vi "ConfigureDifferentialMP.vi"(10 "Right Side":T1, 11 "Left Side":T1) -> (2 "Right Side":T1, 3 "Left Side":T1)   [LabVIEW 2017]
uses:
  <vilib>/Rock Robotics/WPI/MotorControl/WPI_MotorControlDeviceRef.ctl
  <vilib>/Rock Robotics/WPI/MotorControl/WPI_MotorControlType.ctl
  <vilib>/Rock Robotics/SystemInterfaces/DIO/FPGA_DIOPWMChannel.ctl
  <vilib>/Rock Robotics/WPI/PWM/WPI_PWMDeadband.ctl
  <vilib>/Rock Robotics/SystemInterfaces/DIO/FPGA_DIOChannel.ctl
  <vilib>/Rock Robotics/WPI/ThirdParty/Phoenix-LabVIEW/Motor Controller/Controls/CTRE_Phoenix_MotorControl_FeedbackDevice.ctl
  <vilib>/Rock Robotics/WPI/ThirdParty/Phoenix-LabVIEW/Motor Controller/Controls/CTRE_Phoenix_MotorControl_RemoteSourceType.ctl
  <vilib>/Rock Robotics/WPI/ThirdParty/Phoenix-LabVIEW/Motor Controller/Controls/CTRE_Phoenix_MotorControl_SensorTermFeedbackDevice_Enhanced.ctl
  <vilib>/Rock Robotics/WPI/ThirdParty/Phoenix-LabVIEW/Motor Controller/Controls/CTRE_Phoenix_MotorControl_StatusFrameEnhanced.ctl
  <vilib>/Rock Robotics/WPI/ThirdParty/Phoenix-LabVIEW/Motor Controller/Controls/CTRE_Phoenix_MotorControl_NeutralMode.ctl
  <vilib>/Rock Robotics/WPI/ThirdParty/Phoenix-LabVIEW/Motor Controller/Controls/CTRE_Phoenix_MotorControl_ControlMode.ctl
  <vilib>/Rock Robotics/WPI/ThirdParty/Phoenix-LabVIEW/Controls/CTRE_Phoenix_Params.ctl
  Constants.vi
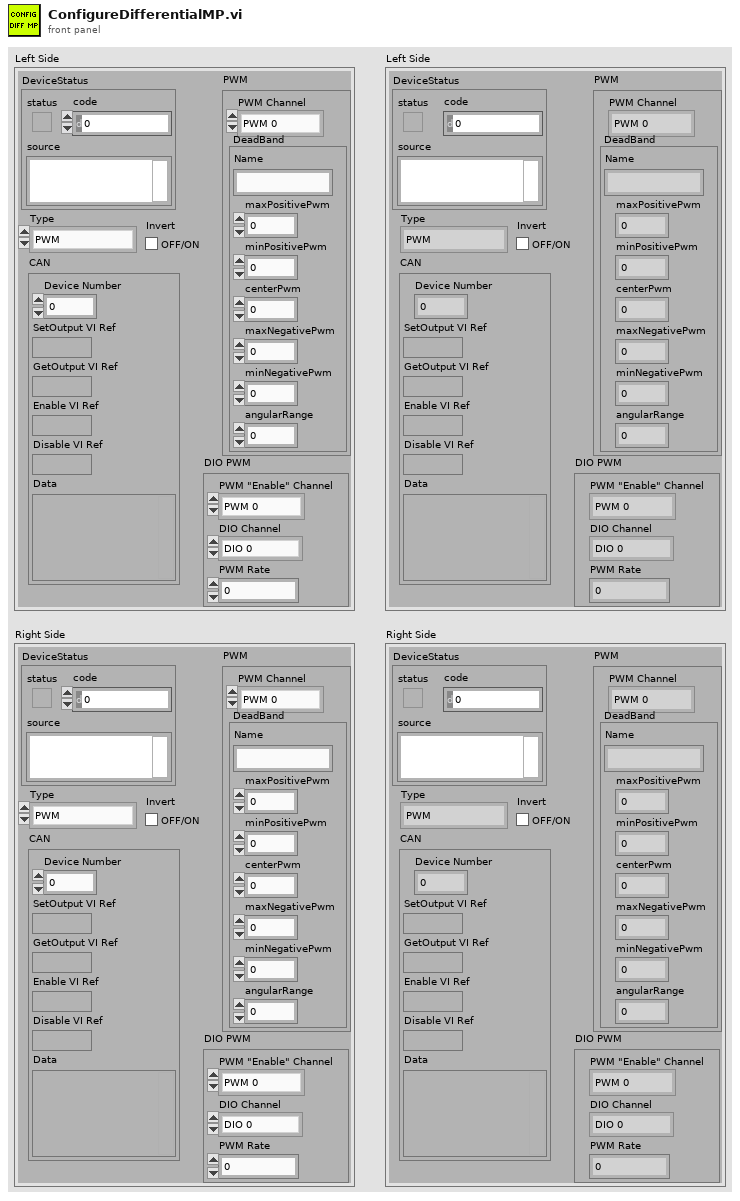
[diagram p1: front panel]
types:
  T1 = typedef "WPI_MotorControlDeviceRef.ctl" = cluster{"DeviceStatus":errorcluster, "Type":T2, "PWM":cluster{"PWM Channel":T3, "DeadBand":T4}, "CAN":cluster{"Device Number":u8, "SetOutput VI Ref":variant, "GetOutput VI Ref":variant, "Enable VI Ref":variant, "Disable VI Ref":variant, "Data":variant}, "Invert":bool, "DIO PWM":cluster{"PWM \"Enable\" Channel":T3, "DIOChannel":T5, "PWM Rate":dbl}}
  T2 = typedef "WPI_MotorControlType.ctl" = enum16{"PWM", "CAN", "DIO PWM"}
  T3 = typedef "FPGA_DIOPWMChannel.ctl" = enum8{"PWM 0", "PWM 1", "PWM 2", "PWM 3", "PWM 4", "PWM 5", "PWM 6", "PWM 7", "PWM 8", "PWM 9", "PWM MXP 0", "PWM MXP 1", "PWM MXP 2", "PWM MXP 3", "PWM MXP 4", "PWM MXP 5", "PWM MXP 6", "PWM MXP 7", "PWM MXP 8", "PWM MXP 9", "Invalid"}
  T4 = typedef "WPI_PWMDeadband.ctl" = cluster{"Name":string, "maxPositivePwm":i32, "minPositivePwm":i32, "centerPwm":i32, "maxNegativePwm":i32, "minNegativePwm":i32, "angularRange":u16}
  T5 = typedef "FPGA_DIOChannel.ctl" = enum8{"DIO 0", "DIO 1", "DIO 2", "DIO 3", "DIO 4", "DIO 5", "DIO 6", "DIO 7", "DIO 8", "DIO 9", "DIO MXP 0", "DIO MXP 1", "DIO MXP 2", "DIO MXP 3", "DIO MXP 4", "DIO MXP 5", "DIO MXP 6", "DIO MXP 7", "DIO MXP 8", "DIO MXP 9", "DIO MXP 10", "DIO MXP 11", "DIO MXP 12", "DIO MXP 13", "DIO MXP 14", "DIO MXP 15", "SPI Port CS1", "SPI Port CS2", "SPI Port CS3", "SPI Port MISO", "SPI Port MOSI", "Invalid"}
  T6 = typedef "CTRE_Phoenix_Params.ctl" = u16
  T7 = typedef "CTRE_Phoenix_MotorControl_ControlMode.ctl" = u16
  T8 = typedef "CTRE_Phoenix_MotorControl_NeutralMode.ctl" = enum8{"EEPROMSetting", "Override to Coast", "Override to Brake"}
  T9 = typedef "CTRE_Phoenix_MotorControl_StatusFrameEnhanced.ctl" = u16
  T10 = typedef "CTRE_Phoenix_MotorControl_FeedbackDevice.ctl" = i8
  T11 = typedef "CTRE_Phoenix_MotorControl_SensorTermFeedbackDevice_Enhanced.ctl" = i8
  T12 = typedef "CTRE_Phoenix_MotorControl_RemoteSourceType.ctl" = enum16{"Off", "Talon SRX Selected Sensor", "Pigeon IMU Yaw", "Pigeon IMU Pitch", "Pigeon IMU Roll", "CANifier Quadrature", "CANifier PWM Input 0", "CANifier PWM Input 1", "CANifier PWM Input 2", "CANifier PWM Input 3", "Gadgeteer Pigeon Yaw", "Gadgeteer Pigeon Pitch", "Gadgeteer Pigeon Roll"}
  T13 = cluster{"kP":dbl, "kI ":dbl, "kD":dbl, "kF":dbl, "I Zone":dbl, "Peak Out":dbl}
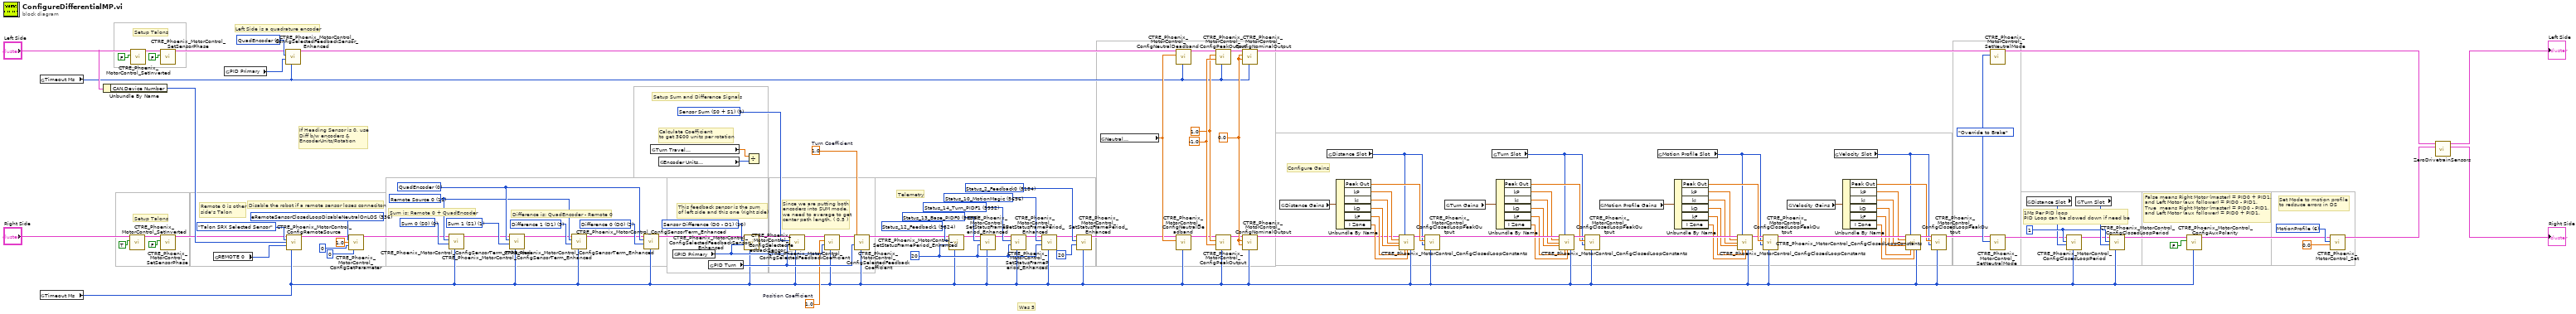
[diagram p0: block diagram]
diagram:
  w1 = 1.0  # Turn Coefficient
  w7 = T6 336 items=["eOnBoot_BrakeMode"=31, "eQuadFilterEn"=91, "eQuadIdxPolarity"=108, "eClearPositionOnIdx"=100, "eMotionProfileHasUnderrunErr"=119, "eMotionProfileTrajectoryPointDurationMs"=120, "eClearPosOnLimitF"=144, "eClearPosOnLimitR"=145, "eStatusFramePeriod"=300, "eOpenLoopRamp"=301, "eClosedLoopRamp"=302, "eNeutralDeadband"=303, "ePeakPosOutput"=305, "eNominalPosOutput"=306, "ePeakNegOutput"=307, "eNominalNegOutput"=308, "eProfileParamSlot_P"=310, "eProfileParamSlot_I"=311, "eProfileParamSlot_D"=312, "eProfileParamSlot_F"=313, "eProfileParamSlot_IZone"=314, "eProfileParamSlot_AllowableErr"=315, "eProfileParamSlot_MaxIAccum"=316, "eClearPositionOnLimitF"=320, "eClearPositionOnLimitR"=321, "eClearPositionOnQuadIdx"=322, "eSampleVelocityPeriod"=325, "eSampleVelocityWindow"=326, "eFeedbackSensorType"=330, "eSelectedSensorPosition"=331, "eFeedbackNotContinuous"=332, "eRemoteSensorSource"=333, "eRemoteSensorDeviceID"=334, "eSensorTerm"=335, "eRemoteSensorClosedLoopDisableNeutralOnLOS"=336, "eForwardSoftLimitThreshold"=340, "eReverseSoftLimitThreshold"=341, "eForwardSoftLimitEnable"=342, "eReverseSoftLimitEnable"=343, "eNominalBatteryVoltage"=350, "eBatterVoltageFilterSize"=351, "eContinuousCurrentLimitAmps"=360, "eContinuousCurrentLimitMs"=361, "ePeakCurrentLimitAmps"=362, "eClosedLoopIAccum"=370, "eCustomParam"=380, "eStickyFaults"=390, "eAnalogPosition"=400, "eQuadraturePosition"=401, "ePulseWidthPosition"=402, "eMotMag_Accel"=410, "eMotMag_VelCruise"=411, "eLimitSwitchSource"=421, "eLimitSwitchNormClosedAndDis"=422, "eLimitSwitchDisabledNeutralOnLOS"=423, "eLimitSwitchRemoteDevID"=424] ("Parameter")
  w20 = T7 6 items=["PercentOutput"=0, "Position"=1, "Velocity"=2, "Current"=3, "Follower"=5, "MotionProfile"=6, "MotionMagic"=7, "MotionProfileArc"=10, "Disabled"=15] ("Control Mode")
  w120 = 1 ("loopTimeMs")
  w116 = CTRE_Phoenix_MotorControl_NeutralMode."Override to Brake" ("Motor Control Neutral Mode")
  w77 = 0.0 ("Forward Nominal Percent Output")
  w74 = -1.0 ("Reverse Peak Percent Output")
  w73 = 1.0 ("Forward Peak Percent Output")
  w16 = 20 ("periodMs")
  w66 = T9 5184 items=["Status_1_General"=5120, "Status_2_Feedback0"=5184, "Status_3_Quadrature"=5248, "Status_4_AinTempVbat"=5312, "Status_6_Misc"=5440, "Status_7_CommStatus"=5504, "Status_8_PulseWidth"=5568, "Status_9_MotProfBuffer"=5632, "Status_10_MotionMagic"=5696, "Status_11_UartGadgeteer"=5760, "Status_12_Feedback1"=5824, "Status_13_Base_PIDF0"=5888, "Status_14_Turn_PIDF1"=5952, "Status_15_FirmwareApiStatus"=6016] ("Status Frame")
  w65 = T9 5696 items=["Status_1_General"=5120, "Status_2_Feedback0"=5184, "Status_3_Quadrature"=5248, "Status_4_AinTempVbat"=5312, "Status_6_Misc"=5440, "Status_7_CommStatus"=5504, "Status_8_PulseWidth"=5568, "Status_9_MotProfBuffer"=5632, "Status_10_MotionMagic"=5696, "Status_11_UartGadgeteer"=5760, "Status_12_Feedback1"=5824, "Status_13_Base_PIDF0"=5888, "Status_14_Turn_PIDF1"=5952, "Status_15_FirmwareApiStatus"=6016] ("Status Frame")
  w64 = T9 5952 items=["Status_1_General"=5120, "Status_2_Feedback0"=5184, "Status_3_Quadrature"=5248, "Status_4_AinTempVbat"=5312, "Status_6_Misc"=5440, "Status_7_CommStatus"=5504, "Status_8_PulseWidth"=5568, "Status_9_MotProfBuffer"=5632, "Status_10_MotionMagic"=5696, "Status_11_UartGadgeteer"=5760, "Status_12_Feedback1"=5824, "Status_13_Base_PIDF0"=5888, "Status_14_Turn_PIDF1"=5952, "Status_15_FirmwareApiStatus"=6016] ("Status Frame")
  w63 = T9 5888 items=["Status_1_General"=5120, "Status_2_Feedback0"=5184, "Status_3_Quadrature"=5248, "Status_4_AinTempVbat"=5312, "Status_6_Misc"=5440, "Status_7_CommStatus"=5504, "Status_8_PulseWidth"=5568, "Status_9_MotProfBuffer"=5632, "Status_10_MotionMagic"=5696, "Status_11_UartGadgeteer"=5760, "Status_12_Feedback1"=5824, "Status_13_Base_PIDF0"=5888, "Status_14_Turn_PIDF1"=5952, "Status_15_FirmwareApiStatus"=6016] ("Status Frame")
  w62 = T9 5824 items=["Status_1_General"=5120, "Status_2_Feedback0"=5184, "Status_3_Quadrature"=5248, "Status_4_AinTempVbat"=5312, "Status_6_Misc"=5440, "Status_7_CommStatus"=5504, "Status_8_PulseWidth"=5568, "Status_9_MotProfBuffer"=5632, "Status_10_MotionMagic"=5696, "Status_11_UartGadgeteer"=5760, "Status_12_Feedback1"=5824, "Status_13_Base_PIDF0"=5888, "Status_14_Turn_PIDF1"=5952, "Status_15_FirmwareApiStatus"=6016] ("Status Frame")
  w53 = 1.0  # Position Coefficient
  w14 = T10 9 items=["None"=-1, "QuadEncoder"=0, "Analog"=2, "Tachometer"=4, "Pulse Width Encoded Position"=8, "Sensor Sum (S0 + S1)"=9, "Sensor Difference (D0 - D1)"=10, "Remote Source 0"=11, "Remote Source 1"=12, "Software Emulated"=15] ("Feedback Device")
  w50 = T10 10 items=["None"=-1, "QuadEncoder"=0, "Analog"=2, "Tachometer"=4, "Pulse Width Encoded Position"=8, "Sensor Sum (S0 + S1)"=9, "Sensor Difference (D0 - D1)"=10, "Remote Source 0"=11, "Remote Source 1"=12, "Software Emulated"=15] ("Feedback Device")
  w48 = u16 2 items=["Sum 0 (S0)", "Sum 1 (S1)", "Difference 0 (D0)", "Difference 1 (D1)"] ("Sensor Term")
  w47 = u16 3 items=["Sum 0 (S0)", "Sum 1 (S1)", "Difference 0 (D0)", "Difference 1 (D1)"] ("Sensor Term")
  w42 = u16 1 items=["Sum 0 (S0)", "Sum 1 (S1)", "Difference 0 (D0)", "Difference 1 (D1)"] ("Sensor Term")
  w46 = T11 0 items=["None"=-1, "QuadEncoder"=0, "Analog"=2, "Tachometer"=4, "Pulse Width Encoded Position"=8, "Remote Source 0"=11, "Remote Source 1"=12, "Software Emulated"=15] ("Feedback Device")
  w40 = u16 0 items=["Sum 0 (S0)", "Sum 1 (S1)", "Difference 0 (D0)", "Difference 1 (D1)"] ("Sensor Term")
  w45 = T11 11 items=["None"=-1, "QuadEncoder"=0, "Analog"=2, "Tachometer"=4, "Pulse Width Encoded Position"=8, "Remote Source 0"=11, "Remote Source 1"=12, "Software Emulated"=15] ("Feedback Device")
  w34 = T10 0 items=["None"=-1, "QuadEncoder"=0, "Analog"=2, "Tachometer"=4, "Pulse Width Encoded Position"=8, "Sensor Sum (S0 + S1)"=9, "Sensor Difference (D0 - D1)"=10, "Remote Source 0"=11, "Remote Source 1"=12, "Software Emulated"=15] ("Feedback Device")
  # "Was 5"
  # "Disable the robot if a remote sensor loses conneciton"
  # "Set Mode to motion profile\nto redsuce errors in DS"
  # "False means Right Motor (master) = PID0 + PID1, \nand Left Motor (aux follower) = PID0 - PID1.\nTrue  means Right Motor (master) = PID0 - PID1, \nand Left Motor (aux follower) = PID0 + PID1."
  # "1Ms Per PID loop\nPID Loop can be slowed down if need be"
  # "Configure Gains"
  # "Setup Talons"
  # "Telemetry"
  # "Since we are putting both\nencoders into SUM mode,\nwe need to average to get\ncenter path length. ( 0.5 )"
  # "Calculate Coefficient\nto get 3600 units per rotation"
  # "If Heading Sensor is 0, use \nDiff b/w encoders &\nEncoderUnits/Rotation"
  # "This feedback sensor is the sum\nof left side and this one (right side)"
  # "Difference is: QuadEncoder - Remote 0"
  # "Sum is: Remote 0 + QuadEncoder"
  # "Setup Sum and Difference Signals"
  # "Remote 0 is other\nside's Talon"
  # "Left Side is a quadrature encoder"
  # "Setup Talons"
  n1 = global read "Constants.vi" "Timeout Ms"() -> (w9:i32)
  n2 = global read "Constants.vi" "Timeout Ms"() -> (w8:i32)
  n3 = Unbundle By Name("Left Side") -> ("CAN.Device Number"=w38:u8)
  n4 = call <vilib>:"CTRE_Phoenix_MotorControl_SetInverted.vi"("Invert?"=TRUE, "PhoenixMotorControlDevRef"="Right Side") -> ("PhoenixMotorControlDevRef"=w30:T1)  [unwired: 8 in, 1 out]
  n5 = call <vilib>:"CTRE_Phoenix_MotorControl_SetInverted.vi"("Invert?"=FALSE, "PhoenixMotorControlDevRef"="Left Side") -> ("PhoenixMotorControlDevRef"=w29:T1)  [unwired: 8 in, 1 out]
  n6 = call <vilib>:"CTRE_Phoenix_MotorControl_SetSensorPhase.vi"("PhaseSensor"=FALSE, "PhoenixMotorControlDevRef"=w29) -> ("PhoenixMotorControlDevRef"=w33:T1)  [unwired: 8 in, 1 out]
  n7 = call <vilib>:"CTRE_Phoenix_MotorControl_SetSensorPhase.vi"("PhaseSensor"=FALSE, "PhoenixMotorControlDevRef"=w30) -> ("PhoenixMotorControlDevRef"=w35:T1)  [unwired: 8 in, 1 out]
  n8 = global read "Constants.vi" "REMOTE 0"() -> (w39:i32)
  n9 = global read "Constants.vi" "PID Primary"() -> (w123:i32)
  n10 = call <vilib>:"CTRE_Phoenix_MotorControl_ConfigSelectedFeedbackSensor_Enhanced.vi"("timeoutMs"=w9, "pidLoopIdx"=w123, "Feedback Device"=w34, "PhoenixMotorControlDevRef"=w33) -> ("PhoenixMotorControlDevRef"=w70:T1)  [unwired: 6 in, 1 out]
  n11 = call <vilib>:"CTRE_Phoenix_MotorControl_ConfigRemoteSource.vi"("PhoenixMotorControlDevRef"=w35, "Remote Device Type"=CTRE_Phoenix_MotorControl_RemoteSourceType."Talon SRX Selected Sensor", "Remote Device ID"=w38, "Source Index (0/1)"=w39, "timeoutMs"=w8) -> ("PhoenixMotorControlDevRef"=w3:T1)  [unwired: 9 in, 1 out]
  n12 = call <vilib>:"CTRE_Phoenix_MotorControl_ConfigSetParameter.vi"("PhoenixMotorControlDevRef"=w3, "Parameter"=w7, "value"=1.0, "subValue"=u8 0, "ordinal"=0) -> ("PhoenixMotorControlDevRef"=w2:T1)  [unwired: 9 in, 1 out]
  n13 = call <vilib>:"CTRE_Phoenix_MotorControl_ConfigSensorTerm_Enhanced.vi"("timeoutMs"=w8, "Sensor Term"=w40, "Feedback Device"=w45, "PhoenixMotorControlDevRef"=w2) -> ("PhoenixMotorControlDevRef"=w41:T1)  [unwired: 6 in, 1 out]
  n14 = call <vilib>:"CTRE_Phoenix_MotorControl_ConfigSensorTerm_Enhanced.vi"("timeoutMs"=w8, "Sensor Term"=w42, "Feedback Device"=w46, "PhoenixMotorControlDevRef"=w41) -> ("PhoenixMotorControlDevRef"=w44:T1)  [unwired: 6 in, 1 out]
  n15 = call <vilib>:"CTRE_Phoenix_MotorControl_ConfigSensorTerm_Enhanced.vi"("timeoutMs"=w8, "Sensor Term"=w47, "Feedback Device"=w45, "PhoenixMotorControlDevRef"=w44) -> ("PhoenixMotorControlDevRef"=w43:T1)  [unwired: 6 in, 1 out]
  n16 = call <vilib>:"CTRE_Phoenix_MotorControl_ConfigSensorTerm_Enhanced.vi"("timeoutMs"=w8, "Sensor Term"=w48, "Feedback Device"=w46, "PhoenixMotorControlDevRef"=w43) -> ("PhoenixMotorControlDevRef"=w49:T1)  [unwired: 6 in, 1 out]
  n17 = global read "Constants.vi" "Turn Travel\nUnits Per Rotation"() -> (w56:dbl)
  n18 = global read "Constants.vi" "Encoder Units\nPer Rotation"() -> (w15:i32)
  n19 = global read "Constants.vi" "PID Primary"() -> (w122:i32)
  n20 = global read "Constants.vi" "PID Turn"() -> (w55:i32)
  n21 = call <vilib>:"CTRE_Phoenix_MotorControl_ConfigSelectedFeedbackSensor_Enhanced.vi"("timeoutMs"=w8, "pidLoopIdx"=w122, "Feedback Device"=w50, "PhoenixMotorControlDevRef"=w49) -> ("PhoenixMotorControlDevRef"=w51:T1)  [unwired: 6 in, 1 out]
  n22 = Divide(x=w56, y=w15) -> ()  [unwired: 1 out]
  n23 = call <vilib>:"CTRE_Phoenix_MotorControl_ConfigSelectedFeedbackSensor_Enhanced.vi"("timeoutMs"=w8, "pidLoopIdx"=w55, "Feedback Device"=w14, "PhoenixMotorControlDevRef"=w51) -> ("PhoenixMotorControlDevRef"=w52:T1)  [unwired: 6 in, 1 out]
  n24 = call <vilib>:"CTRE_Phoenix_MotorControl_ConfigSelectedFeedbackCoefficient.vi"("timoutMs"=w8, "pidIdx"=w122, "coefficient"=w53, "PhoenixMotorControlDevRef"=w52) -> ("PhoenixMotorControlDevRef"=w54:T1)  [unwired: 6 in, 1 out]
  n25 = call <vilib>:"CTRE_Phoenix_MotorControl_ConfigSelectedFeedbackCoefficient.vi"("timoutMs"=w8, "pidIdx"=w55, "coefficient"=w1, "PhoenixMotorControlDevRef"=w54) -> ("PhoenixMotorControlDevRef"=w57:T1)  [unwired: 6 in, 1 out]
  n26 = call <vilib>:"CTRE_Phoenix_MotorControl_SetStatusFramePeriod_Enhanced.vi"("timeoutMs"=w8, "periodMs"=w16, "Status Frame"=w62, "PhoenixMotorControlDevRef"=w57) -> ("PhoenixMotorControlDevRef"=w58:T1)  [unwired: 6 in, 1 out]
  n27 = call <vilib>:"CTRE_Phoenix_MotorControl_SetStatusFramePeriod_Enhanced.vi"("timeoutMs"=w8, "periodMs"=w16, "Status Frame"=w63, "PhoenixMotorControlDevRef"=w58) -> ("PhoenixMotorControlDevRef"=w59:T1)  [unwired: 6 in, 1 out]
  n28 = call <vilib>:"CTRE_Phoenix_MotorControl_SetStatusFramePeriod_Enhanced.vi"("timeoutMs"=w8, "periodMs"=w16, "Status Frame"=w64, "PhoenixMotorControlDevRef"=w59) -> ("PhoenixMotorControlDevRef"=w60:T1)  [unwired: 6 in, 1 out]
  n29 = call <vilib>:"CTRE_Phoenix_MotorControl_SetStatusFramePeriod_Enhanced.vi"("timeoutMs"=w8, "periodMs"=w16, "Status Frame"=w65, "PhoenixMotorControlDevRef"=w60) -> ("PhoenixMotorControlDevRef"=w61:T1)  [unwired: 6 in, 1 out]
  n30 = call <vilib>:"CTRE_Phoenix_MotorControl_SetStatusFramePeriod_Enhanced.vi"("timeoutMs"=w8, "periodMs"=20, "Status Frame"=w66, "PhoenixMotorControlDevRef"=w61) -> ("PhoenixMotorControlDevRef"=w68:T1)  [unwired: 6 in, 1 out]
  n31 = global read "Constants.vi" "Neutral\nDeadband"() -> (w71:dbl)
  n32 = call <vilib>:"CTRE_Phoenix_MotorControl_ConfigNeutralDeadband.vi"("timeoutMs"=w9, "Percent Deadband"=w71, "PhoenixMotorControlDevRef"=w70) -> ("PhoenixMotorControlDevRef"=w72:T1)  [unwired: 7 in, 1 out]
  n33 = call <vilib>:"CTRE_Phoenix_MotorControl_ConfigNeutralDeadband.vi"("timeoutMs"=w8, "Percent Deadband"=w71, "PhoenixMotorControlDevRef"=w68) -> ("PhoenixMotorControlDevRef"=w69:T1)  [unwired: 7 in, 1 out]
  n34 = call <vilib>:"CTRE_Phoenix_MotorControl_ConfigPeakOutput.vi"("timeoutMs"=w9, "Reverse Peak Percent Output"=w74, "Forward Peak Percent Output"=w73, "PhoenixMotorControlDevRef"=w72) -> ("PhoenixMotorControlDevRef"=w76:T1)  [unwired: 6 in, 1 out]
  n35 = call <vilib>:"CTRE_Phoenix_MotorControl_ConfigPeakOutput.vi"("timeoutMs"=w8, "Reverse Peak Percent Output"=w74, "Forward Peak Percent Output"=w73, "PhoenixMotorControlDevRef"=w69) -> ("PhoenixMotorControlDevRef"=w75:T1)  [unwired: 6 in, 1 out]
  n36 = call <vilib>:"CTRE_Phoenix_MotorControl_ConfigNominalOutput.vi"("timeoutMs"=w9, "Reverse Nominal Percent Output"=w77, "Forward Nominal Percent Output"=w77, "PhoenixMotorControlDevRef"=w76) -> ("PhoenixMotorControlDevRef"=w115:T1)  [unwired: 6 in, 1 out]
  n37 = call <vilib>:"CTRE_Phoenix_MotorControl_ConfigNominalOutput.vi"("timeoutMs"=w8, "Reverse Nominal Percent Output"=w77, "Forward Nominal Percent Output"=w77, "PhoenixMotorControlDevRef"=w75) -> ("PhoenixMotorControlDevRef"=w78:T1)  [unwired: 6 in, 1 out]
  n38 = global read "Constants.vi" "Distance Gains"() -> (w79:T13)
  n39 = global read "Constants.vi" "Distance Slot"() -> (w23:i32)
  n40 = Unbundle By Name(w79) -> ("Peak Out"=w86:dbl, "kP"=w80:dbl, "kI"=w81:dbl, "kD"=w82:dbl, "kF"=w83:dbl, "I Zone"=w84:dbl)
  n41 = call <vilib>:"CTRE_Phoenix_MotorControl_ConfigClosedLoopConstants.vi"("PhoenixMotorControlDevRef"=w78, "slotIdx"=w23, "P"=w80, "I"=w81, "D"=w82, "F"=w83, "I Zone"=w84, "timeoutMs"=w8) -> ("PhoenixMotorControlDevRef"=w85:T1)  [unwired: 6 in, 1 out]
  n42 = call <vilib>:"CTRE_Phoenix_MotorControl_ConfigClosedLoopPeakOutput.vi"("timoutMs"=w8, "slotIdx"=w23, "peakOutput"=w86, "PhoenixMotorControlDevRef"=w85) -> ("PhoenixMotorControlDevRef"=w111:T1)  [unwired: 6 in, 1 out]
  n43 = global read "Constants.vi" "Turn Gains"() -> (w94:T13)
  n44 = global read "Constants.vi" "Turn Slot"() -> (w22:i32)
  n45 = Unbundle By Name(w94) -> ("Peak Out"=w87:dbl, "kP"=w93:dbl, "kI"=w92:dbl, "kD"=w91:dbl, "kF"=w90:dbl, "I Zone"=w89:dbl)
  n46 = call <vilib>:"CTRE_Phoenix_MotorControl_ConfigClosedLoopConstants.vi"("PhoenixMotorControlDevRef"=w111, "slotIdx"=w22, "P"=w93, "I"=w92, "D"=w91, "F"=w90, "I Zone"=w89, "timeoutMs"=w8) -> ("PhoenixMotorControlDevRef"=w88:T1)  [unwired: 6 in, 1 out]
  n47 = call <vilib>:"CTRE_Phoenix_MotorControl_ConfigClosedLoopPeakOutput.vi"("timoutMs"=w8, "slotIdx"=w22, "peakOutput"=w87, "PhoenixMotorControlDevRef"=w88) -> ("PhoenixMotorControlDevRef"=w112:T1)  [unwired: 6 in, 1 out]
  n48 = global read "Constants.vi" "Motion Profile Gains"() -> (w95:T13)
  n49 = global read "Constants.vi" "Motion Profile Slot"() -> (w24:i32)
  n50 = Unbundle By Name(w95) -> ("Peak Out"=w102:dbl, "kP"=w96:dbl, "kI"=w97:dbl, "kD"=w98:dbl, "kF"=w99:dbl, "I Zone"=w100:dbl)
  n51 = call <vilib>:"CTRE_Phoenix_MotorControl_ConfigClosedLoopConstants.vi"("PhoenixMotorControlDevRef"=w112, "slotIdx"=w24, "P"=w96, "I"=w97, "D"=w98, "F"=w99, "I Zone"=w100, "timeoutMs"=w8) -> ("PhoenixMotorControlDevRef"=w101:T1)  [unwired: 6 in, 1 out]
  n52 = call <vilib>:"CTRE_Phoenix_MotorControl_ConfigClosedLoopPeakOutput.vi"("timoutMs"=w8, "slotIdx"=w24, "peakOutput"=w102, "PhoenixMotorControlDevRef"=w101) -> ("PhoenixMotorControlDevRef"=w113:T1)  [unwired: 6 in, 1 out]
  n53 = global read "Constants.vi" "Velocity Gains"() -> (w110:T13)
  n54 = global read "Constants.vi" "Velocity Slot"() -> (w21:i32)
  n55 = Unbundle By Name(w110) -> ("Peak Out"=w103:dbl, "kP"=w109:dbl, "kI"=w108:dbl, "kD"=w107:dbl, "kF"=w106:dbl, "I Zone"=w105:dbl)
  n56 = call <vilib>:"CTRE_Phoenix_MotorControl_ConfigClosedLoopConstants.vi"("PhoenixMotorControlDevRef"=w113, "slotIdx"=w21, "P"=w109, "I"=w108, "D"=w107, "F"=w106, "I Zone"=w105, "timeoutMs"=w8) -> ("PhoenixMotorControlDevRef"=w104:T1)  [unwired: 6 in, 1 out]
  n57 = call <vilib>:"CTRE_Phoenix_MotorControl_ConfigClosedLoopPeakOutput.vi"("timoutMs"=w8, "slotIdx"=w21, "peakOutput"=w103, "PhoenixMotorControlDevRef"=w104) -> ("PhoenixMotorControlDevRef"=w114:T1)  [unwired: 6 in, 1 out]
  n58 = call <vilib>:"CTRE_Phoenix_MotorControl_SetNeutralMode.vi"("Motor Control Neutral Mode"=w116, "PhoenixMotorControlDevRef"=w115) -> ("PhoenixMotorControlDevRef"=w13:T1)  [unwired: 8 in, 1 out]
  n59 = call <vilib>:"CTRE_Phoenix_MotorControl_SetNeutralMode.vi"("Motor Control Neutral Mode"=w116, "PhoenixMotorControlDevRef"=w114) -> ("PhoenixMotorControlDevRef"=w117:T1)  [unwired: 8 in, 1 out]
  n60 = global read "Constants.vi" "Distance Slot"() -> (w118:i32)
  n61 = call <vilib>:"CTRE_Phoenix_MotorControl_ConfigClosedLoopPeriod.vi"("timoutMs"=w8, "slotIdx"=w118, "loopTimeMs"=w120, "PhoenixMotorControlDevRef"=w117) -> ("PhoenixMotorControlDevRef"=w119:T1)  [unwired: 6 in, 1 out]
  n62 = global read "Constants.vi" "Turn Slot"() -> (w121:i32)
  n63 = call <vilib>:"CTRE_Phoenix_MotorControl_ConfigClosedLoopPeriod.vi"("timoutMs"=w8, "slotIdx"=w121, "loopTimeMs"=w120, "PhoenixMotorControlDevRef"=w119) -> ("PhoenixMotorControlDevRef"=w26:T1)  [unwired: 6 in, 1 out]
  n64 = call <vilib>:"CTRE_Phoenix_MotorControl_ConfigAuxPolarity.vi"("timeoutMs"=w8, "Invert"=FALSE, "PhoenixMotorControlDevRef"=w26) -> ("PhoenixMotorControlDevRef"=w18:T1)  [unwired: 8 in]
  n65 = call <vilib>:"CTRE_Phoenix_MotorControl_Set.vi"("Output"=0.0, "Control Mode"=w20, "PhoenixMotorControlDevRef"=w18) -> ("PhoenixMotorControlDevRef"=w12:T1)  [unwired: 7 in, 1 out]
  n66 = call "ZeroDrivetrainSensors.vi"("Talon 2"=w12, "Talon 1"=w13) -> ("Talon 2"=→"Right Side":T1, "Talon 1"=→"Left Side":T1)  [unwired: 8 in]
